vi "TRITON_ARRAY_REGISTER.vi"(1 "Input array":dbl[](array[numeric]), 2 "New value":dbl) -> (0 "Updated array":dbl[](array[numeric]))   [LabVIEW 2009]
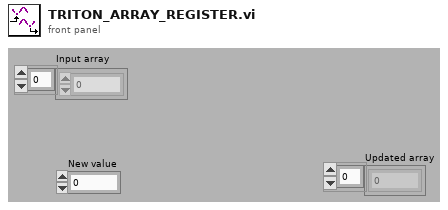
[diagram p1: front panel]
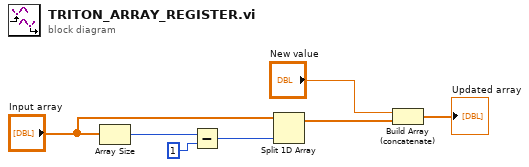
[diagram p0: block diagram]
diagram:
  n1 = Array Size(array="Input array") -> (size(s)=w7:i32)
  n2 = Subtract(x=w7, y=1) -> (x-y=w5:i32)
  n3 = Split 1D Array(array="Input array", index=w5) -> (first subarray=w2:dbl[])  [unwired: 1 out]
  n4 = Build Array (concatenate)("New value", w2) -> (→"Updated array":dbl[])
